vi "XW_Map_Wrapper test_Polysurf_PN.vi"() -> ()   [LabVIEW 2011]
uses:
  XW_Map_Global.vi
panel:
  in  "Apply calib. corrections":bool
  in  "n2 from Vel. Calib":dbl=0.41
  in  "B2 from Vel. Calib":dbl=1.4
  in  "A2 from Vel. Calib":dbl=2.25
  in  "n1 from Vel. Calib":dbl=0.42
  in  "B1 from Vel. Calib":dbl=1.36
  in  "A1 from Vel. Calib":dbl=2.21
  out "st. dev. in abs. % err in Ucal":dbl=2.483081027530719 format="%.6f"
  out "mean abs. % err in Ucal":dbl=1.525679410168452 format="%.6f"
  in  "file path (dialog if empty)":path=path "C:/Documents and Settings/Paul Nathan/Desktop/XW Calib Map/XW Calib Map POLYSURF vi/XW_Map_Wire001OH65_080210.txt"
  out "V (m/s)":dbl=2.620455465537373 format="%.6f"
  out "U (m/s)":dbl=8.5593413234246 format="%.6f"
  in  "cap indicial sum to n":bool=TRUE
  in  "surface order (n)":i32=5
  in  "E2 / G2 + O2":dbl=2.2
  in  "E1 / G1 + O1":dbl=2.4
  # "Paul Nathan 02/02/10"
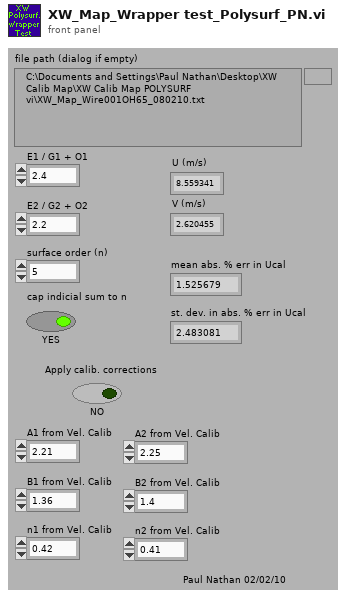
[diagram p1: front panel]
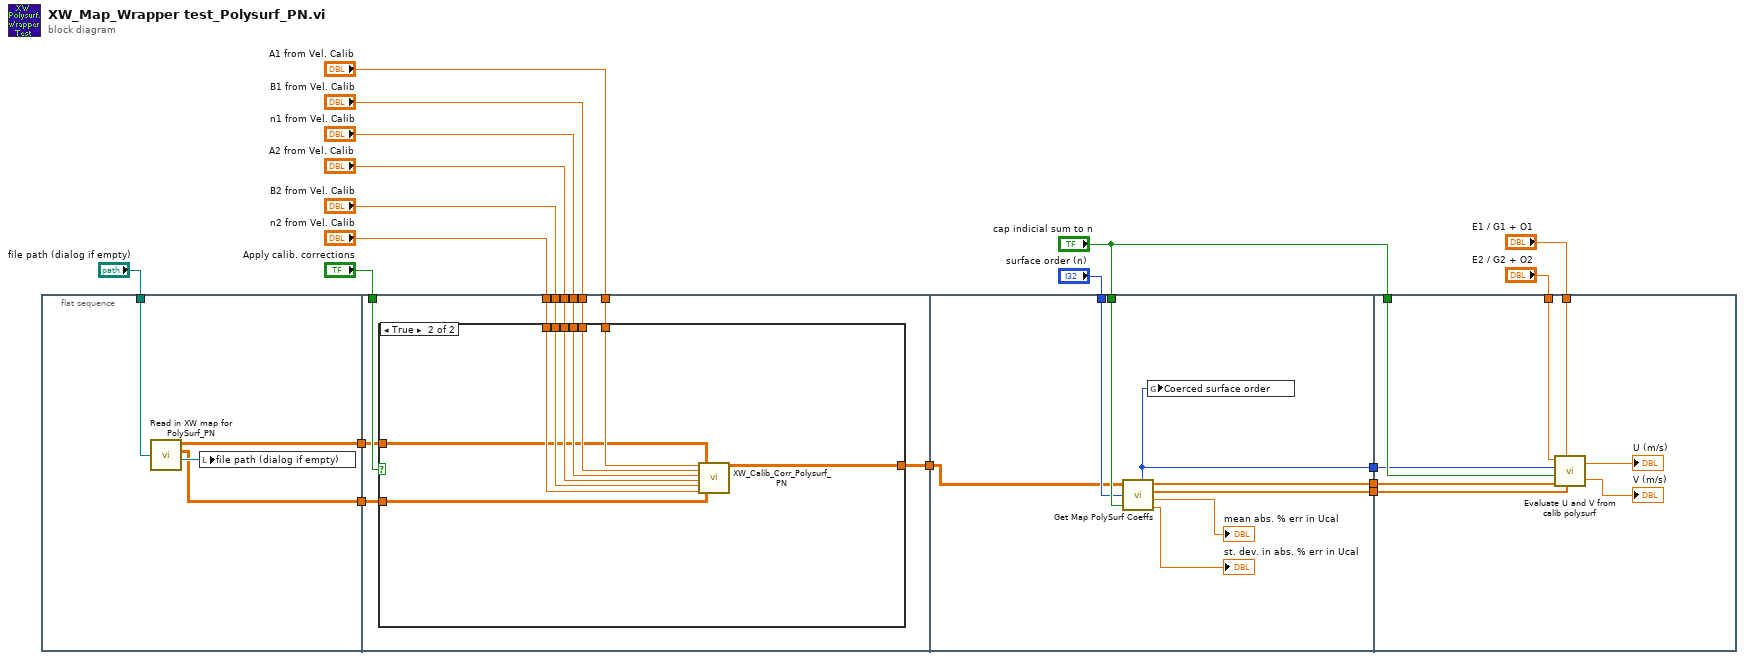
[diagram p0: block diagram]
diagram:
  n1 = flat-sequence {
    tunnel: "file path (dialog if empty)" -> [w22]
    tunnel: [w20] -> w6
    tunnel: [w19] -> w5
    tunnel: "n2 from Vel. Calib" -> [w32]
    tunnel: "B2 from Vel. Calib" -> [w31]
    tunnel: "A2 from Vel. Calib" -> [w30]
    tunnel: "n1 from Vel. Calib" -> [w29]
    tunnel: "B1 from Vel. Calib" -> [w28]
    tunnel: "A1 from Vel. Calib" -> [w27]
    tunnel: "Apply calib. corrections" -> [w26]
    tunnel: w6 -> [w25]
    tunnel: w5 -> [w24]
    tunnel: [w23] -> w4
    tunnel: "cap indicial sum to n" -> [w48]
    tunnel: "surface order (n)" -> [w47]
    tunnel: w4 -> [w46]
    tunnel: [w45] -> w3
    tunnel: [w44] -> w2
    tunnel: [w43] -> w1
    tunnel: "cap indicial sum to n" -> [w56]
    tunnel: "E1 / G1 + O1" -> [w55]
    tunnel: "E2 / G2 + O2" -> [w54]
    tunnel: w3 -> [w53]
    tunnel: w2 -> [w52]
    tunnel: w1 -> [w51]
    frame #0 {
      n2 = call "Read in XW map for PolySurf_PN.vi"("XW map file path (dialog if empty)"=w22) -> ("XW map values"=w20:dbl[][], "Zero angle dataset from map (used for calib. correction)"=w19:dbl[][], "XW map file path"=w21:path)  [unwired: 1 out]
      n3 = local write "file path (dialog if empty)"(w21) -> ()
    }
    frame #1 {
      n4 = case shown="True" w26 {
        tunnel: w32 -> [_ w37]
        tunnel: w31 -> [_ w38]
        tunnel: w30 -> [_ w39]
        tunnel: w29 -> [_ w40]
        tunnel: w28 -> [_ w41]
        tunnel: w27 -> [_ w42]
        tunnel: w25 -> [w33 w36]
        tunnel: w24 -> [_ w35]
        tunnel: [w33 w34] -> w23
        frame False {
        }
        frame True {
          n5 = call "XW_Calib_Corr_Polysurf_PN.vi"("A1 from Vel. Calib"=w42, "B1 from Vel. Calib"=w41, "n1 from Vel. Calib"=w40, "A2 from Vel. Calib"=w39, "B2 from Vel. Calib"=w38, "n2 from Vel. Calib"=w37, "Original XW map values"=w36, "Zero angle dataset from map (used for calib. correction)"=w35) -> ("Corrected XW map values"=w34:dbl[][])  [unwired: 11 out]
        }
      }
    }
    frame #2 {
      n6 = call "Get Map PolySurf Coeffs.vi"("Corrected XW map values"=w46, "surface order (n)"=w47, "cap indicial sum to n"=w48) -> ("Ucal(m/s) coeffs"=w45:dbl[], "alpha(rad) coeffs"=w44:dbl[], "mean abs. % err in Ucal"=→"mean abs. % err in Ucal":dbl, "st. dev. in abs. % err in Ucal"=→"st. dev. in abs. % err in Ucal":dbl, "coerced surface order"=w43:i32)
      n7 = global write "XW_Map_Global.vi" "Coerced surface order"(w43) -> ()
    }
    frame #3 {
      n8 = call "Evaluate U and V from calib polysurf.vi"("alpha(rad) coeffs"=w52, "E1 / G1 + O1"=w55, "Ucal coeffs"=w53, "cap indicial sum to n"=w56, "surface order (n)"=w51, "E2 / G2 + O2"=w54) -> ("V (m/s)"=→"V (m/s)":dbl, "U (m/s)"=→"U (m/s)":dbl)
    }
  }
